vi "HXG2_SavePath.vi"(8 "error in (no error)":errorcluster, 10 "File Name":path, 11 "Folder Name":path) -> (0 "error out":errorcluster, 1 "Base Path":path, 2 "Folder Path":path, 3 "File path":path)   [LabVIEW 2012]
uses:
  <vilib>/Utility/sysdir.llb/System Directory Type.ctl
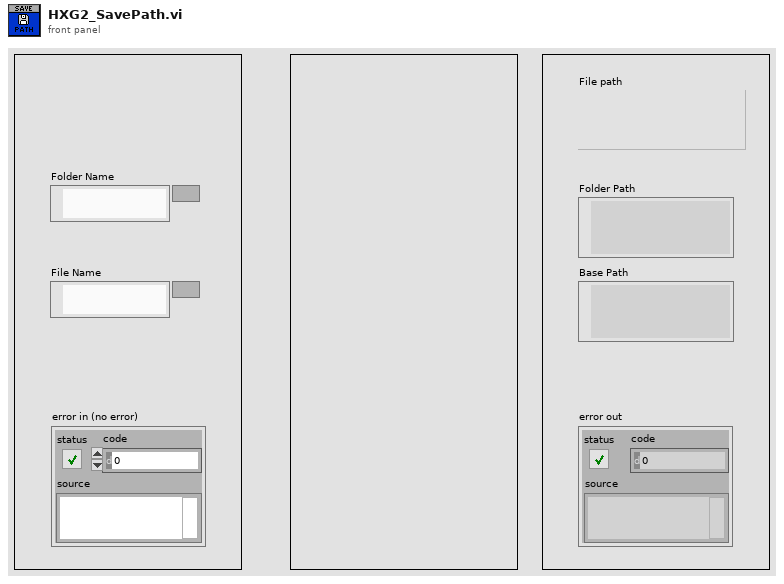
[diagram p1: front panel]
types:
  T1 = typedef "System Directory Type.ctl" = i32
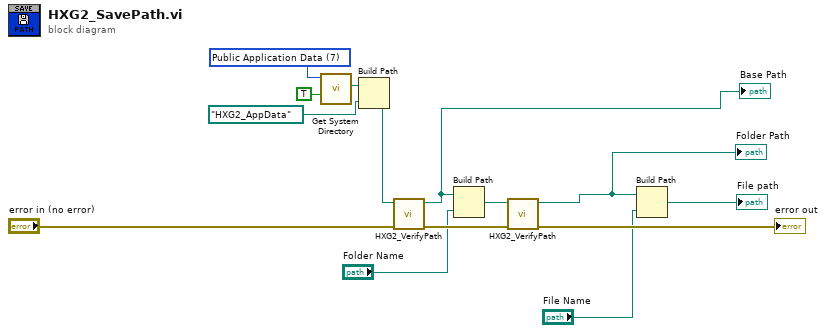
[diagram p0: block diagram]
diagram:
  w7 = T1 7 items=["User Home"=0, "User Desktop"=1, "User Documents"=2, "User Application Data"=3, "User Preferences"=4, "User Temporary"=5, "Public Documents"=6, "Public Application Data"=7, "Public Preferences"=8, "Public Cache"=13, "System Core Libraries"=9, "System Installed Libraries"=10, "Application Files"=11, "Boot Volume Root"=12] ("system directory type")
  n1 = call <vilib>:"Get System Directory.vi"("create directory if not found? (F)"=TRUE, "system directory type"=w7) -> ("system directory"=w9:path)  [unwired: 9 in]
  n2 = Build Path(base path=w9, name or relative path=path "HXG2_AppData" ("Path In")) -> (appended path=w5:path)
  n3 = call "HXG2_VerifyPath.vi"("error in (no error)"="error in (no error)", "Path In"=w5) -> ("error out"=w2:errorcluster, "Path Out"=w11:path)  [unwired: 8 in]
  "Base Path" <- w11
  n4 = Build Path(base path=w11, name or relative path="Folder Name") -> (appended path=w3:path)
  n5 = call "HXG2_VerifyPath.vi"("error in (no error)"=w2, "Path In"=w3) -> ("error out"=→"error out":errorcluster, "Path Out"=w10:path)  [unwired: 8 in]
  "Folder Path" <- w10
  n6 = Build Path(base path=w10, name or relative path="File Name") -> (appended path=→"File path":path)
